vi "Set SPAN for Gasnumber Settings.vi"(7 "set Tables":bool, 8 "error in (no error)":errorcluster caption="Fehler (Eingang, kein Fehler)", 9 "Component Index":i32, 10 "SPNA index":i32, 11 "Digital (Eingang)":refnum<vi>) -> (0 "error out":errorcluster)   [LabVIEW 2020, in "Linearisierung v2.lvlib" / "SpanEinstellungen.lvlib"]
uses:
  SpanEinstellungen.lvlib
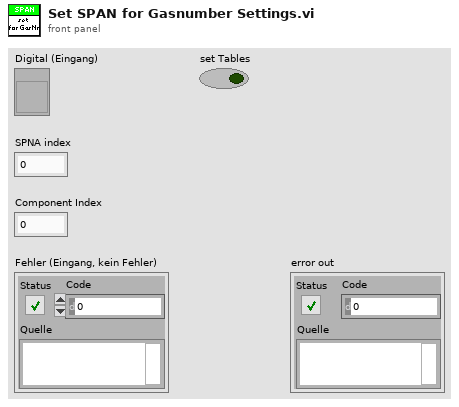
[diagram p1: front panel]
types:
  T1 = cluster{"Komponente:":u16, "Konzentration IST":dbl}[]
  T2 = typedef "Linearisierung v2.lvlib/Gasnumber.ctl" = u8
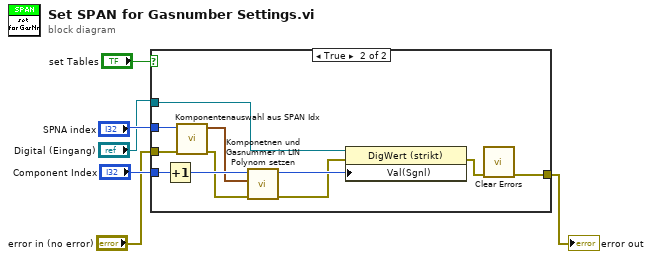
[diagram p0: block diagram]
diagram:
  n1 = case shown="True" "set Tables" {
    tunnel: "Component Index" -> [_ w18]
    tunnel: "SPNA index" -> [_ w14]
    tunnel: "Digital (Eingang)" -> [_ w12]
    tunnel: [w7 w10] -> w2
    tunnel: "error in (no error)" -> [w7 w9]
    frame False {
    }
    frame True {
      n2 = Increment(x=w18) -> (x+1=w16:i32)
      n3 = call "Komponentenauswahl aus SPAN Idx.vi"("Fehler (Eingang, kein Fehler)"=w9, "Span Iindex"=w14) -> ("Fehler (Ausgang)"=w13:errorcluster, "Komponentenauswahl"=w8:T1)  [unwired: 8 in]
      n4 = call "Komponetnen und Gasnummer in LIN Polynom setzen.vi"("Fehler (Eingang, kein Fehler)"=w13, "Komponentenauswahl"=w8, "Gasnummer"=w16) -> ("Fehler (Ausgang)"=w11:errorcluster, "Gasnummer out"=w15:T2)  [unwired: 6 in, 1 out]
      n5 = property on="Eigenschaftsknoten" class="DigWert (strikt)"(reference=w12, error in=w11, "Val(Sgnl)"=w15) -> (error out=w17:errorcluster)  [unwired: 1 out]
      n6 = call <vilib>:"Clear Errors.vi"("error in (no error)"=w17) -> ("error out"=w10:errorcluster)  [unwired: 5 in, 1 out]
    }
  }
  "error out" <- w2
